vi "SL TAGS SystemLink Type To Class.vi"(8 "error in (no error)":errorcluster, 9 "SystemLink Cluster":T7, 11 "Class Tag In":T1={"Class Properties"={"Class Data Type"=enum."Double", "Name"="", "Description"="", "Interpolation Method"=enum."linear", "Unit of Measure"=enum."Hour", "Maximum Interpolation"="", "Role"=enum."Supervisor"}, "SL Tag"=refnum, "SystemLink Cluster"={"Path"="", "Data Type"=enum."Double", "Value"=variant, "Time Stamp"=timestamp(0 s since 1904-01-01)}, "Class Value"=variant}) -> (0 "error out":errorcluster, 3 "Class Tag Out":T1={"Class Properties"={"Class Data Type"=enum."Double", "Name"="", "Description"="", "Interpolation Method"=enum."linear", "Unit of Measure"=enum."Hour", "Maximum Interpolation"="", "Role"=enum."Supervisor"}, "SL Tag"=refnum, "SystemLink Cluster"={"Path"="", "Data Type"=enum."Double", "Value"=variant, "Time Stamp"=timestamp(0 s since 1904-01-01)}, "Class Value"=variant})   [LabVIEW 2017, in "EEISysLink.lvclass"]
doc: "At time of this library development SystemLink has mixed or no support for booleans & waveforms. This VI translates an extended set of data types in the class and more restricted in the SystemLink server from SystemLink type to class type.\n\nThis is a good location to seperate data types in SystemLink from those in the class. This allows the class to support any number of data types and translate to SystemLink types. This class translation is a good candidate for extending with additional data type classes to support an extended library functionality. \n\nJames Tillett P.E.\nEndeavor Engineering Inc.\nwww.endeavoreng.com"
uses:
  EEISysLink.lvclass
  <vilib>/Skyline/Tag/Shared/typedefs/Tag Cluster.ctl
  <vilib>/Skyline/Tag/Shared/typedefs/DataType.ctl
  Controls/SL Tag.ctl
  <vilib>/Skyline/Tag/Wrapper/Wrapper_class/NI Skyline Tag.lvclass
  Controls/SL Tag Properties.ctl
  Controls/SL Tag Data Type.ctl
  Controls/SL Tag Interpolation Method.ctl
  Controls/SL Tag Unit of Measure.ctl
  Controls/SL Tag Type.ctl
  Controls/SL Waveform.ctl
  <vilib>/Skyline/Tag/Shared/NI Skyline Tag.lvlib
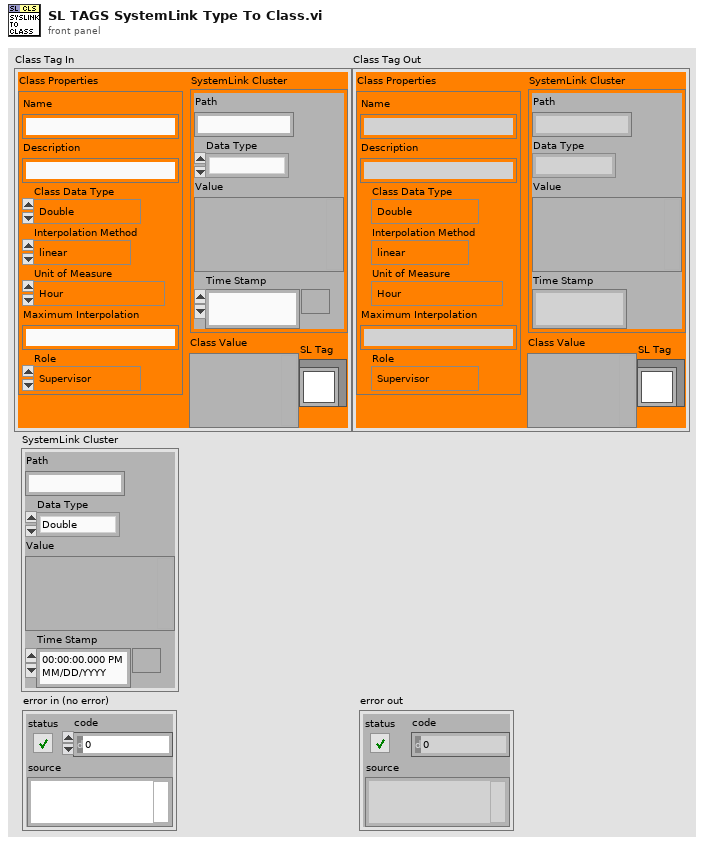
[diagram p1: front panel]
types:
  T1 = typedef "EEISysLink.lvclass/SL Tag.ctl" = cluster{"Class Properties":T2, "SL Tag":refnum<class "NI Skyline Tag.lvclass">, "SystemLink Cluster":T7, "Class Value":variant}
  T2 = typedef "EEISysLink.lvclass/SL Tag Properties.ctl" = cluster{"Class Data Type":T3, "Name":string, "Description":string, "Interpolation Method":T4, "Unit of Measure":T5, "Maximum Interpolation":string, "Role":T6}
  T3 = typedef "EEISysLink.lvclass/SL Tag Data Type.ctl" = enum16{"Double", "Integer", "String", "Boolean", "Waveform"}
  T4 = typedef "EEISysLink.lvclass/SL Tag Interpolation Method.ctl" = enum16{"linear", "pilinear", "step"}
  T5 = typedef "EEISysLink.lvclass/SL Tag Unit of Measure.ctl" = enum16{"no units", "Second", "Hour", "Minute", "Day", "Year", "Month", "Week", "Foot", "Yard", "Meter", "Centimeter", "Inch", "Mile", "Nautical Mile", "Miles per Hour", "Meters per second", "Square meter", "Cubic meter", "Cubic centimeter", "Cubic inch", "Liter", "Gallon", "Gallons dry US", "Gallon UK", "Percent", "Revolutions per minute", "Revolution", "Degree angle", "Astronomical Unit", "Atom", "Atomic mass", "Bar", "Byte", "C (speed of light)", "Curie", "Decibel", "Electron Volt", "Ounce", "Knot", "G", "Grade", "Are", "Hectare", "Faraday", "Franklin", "Gilbert", "Erg", "Lambert", "Maxwell", "Gauss", "Electron mass", "Kilogram force", "Pound force", "Rad", "Centiradian", "Sphere", "Mach", "Fluid Ounces", "Fluid Ounces UK", "Fahrenheit", "Celsius", "Kelvin", "Rankine", "Gram", "Kilogram", "Pound", "Short/US Ton", "Long/UK ton", "Metric ton", "Mole", "Pounds per square inch", "Inches water column", "Torr", "Millitorr", "Millimeter mercury", "Inches mercury", "Bar (2)", "Atmosphere", "Pascal", "Watt", "kiloWatt", "Horsepower", "Kilowatt Hour", "British thermal units", "Millions of BTU", "Ampere", "Candela", "Radian", "Steradian", "Bit", "Hertz", "Newton", "Joule", "Coulomb", "Volt", "Farad", "Ohm", "Siemens", "Weber", "Tesla", "Henry", "Lumen", "Lux", "Becqueral", "Gray", "Sievert", "Katal", "Angstrom", "Light Year", "Parsec", "Point", "Pixel", "Dyne", "Kilogram force (2)", "Pound force (2)", "Rem", "Rutherford", "Roentgen"}
  T6 = typedef "EEISysLink.lvclass/SL Tag Type.ctl" = enum16{"All", "Supervisor", "Worker"}
  T7 = typedef "NI Skyline Tag.lvlib/Tag Cluster.ctl" = cluster{"Path":string, "Data Type":T8, "Value":variant, "Time Stamp":timestamp}
  T8 = typedef "NI Skyline Tag.lvlib/DataType.ctl" = enum32{"Double", "Integer", "String"}
  T9 = typedef "EEISysLink.lvclass/SL Waveform.ctl" = cluster{"t0":dbl, "dt":dbl, "Y":dbl[]}
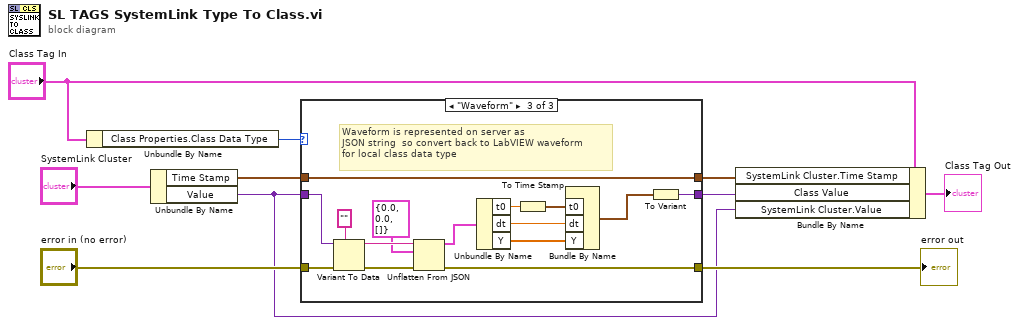
[diagram p0: block diagram]
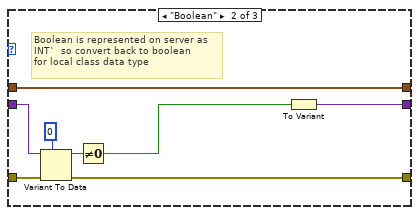
[diagram p3: hidden frame]
diagram:
  n1 = Unbundle By Name("Class Tag In") -> ("Class Properties.Class Data Type"=w10:T3)
  n2 = Unbundle By Name("SystemLink Cluster") -> ("Time Stamp"=w9:timestamp, "Value"=w1:variant)
  n3 = case shown="\"Waveform\"" w10 {
    tunnel: w9 -> [w13 w19 w35]
    tunnel: w1 -> [w12 w21 w36]
    tunnel: [w12 w20 w33] -> w5
    tunnel: [w13 w19 w35] -> w6
    tunnel: "error in (no error)" -> [w11 w18 w34]
    tunnel: [w11 w14 w22] -> w3
    frame Default {
      # "SystemLink supported so pass through unchanged"
    }
    frame "Boolean" {
      # "Boolean is represented on server as \nINT`  so convert back to boolean\nfor local class data type"
      n4 = Variant To Data(error in=w18, type=0, Variant=w21) -> (data=w16:i32, error out=w14:errorcluster)
      n5 = Not Equal To 0?(x=w16) -> (x != 0?=w15:bool)
      n6 = To Variant(anything=w15) -> (Variant=w20:variant)
    }
    frame "Waveform" {
      # "Waveform is represented on server as \nJSON string  so convert back to LabVIEW waveform\nfor local class data type"
      n7 = Variant To Data(error in=w34, type="", Variant=w36) -> (data=w30:string, error out=w31:errorcluster)
      n8 = Unflatten From JSON(JSON string=w30, type and defaults=T9 {"t0"=0.0, "dt"=0.0, "Y"=[]} ("SL Waveform"), error in (no error)=w31) -> (value=w28:T9, error out=w22:errorcluster)  [unwired: 4 in]
      n9 = Unbundle By Name(w28) -> ("t0"=w27:dbl, "dt"=w25:dbl, "Y"=w24:dbl[])
      n10 = To Time Stamp(1:w27) -> (0:w26:timestamp)
      n11 = Bundle By Name("t0"=w26, "dt"=w25, "Y"=w24) -> (w23:waveform(dbl))  [unwired: 1 in]
      n12 = To Variant(anything=w23) -> (Variant=w33:variant)
    }
  }
  "error out" <- w3
  n13 = Bundle By Name(cluster="Class Tag In", "SystemLink Cluster.Time Stamp"=w6, "Class Value"=w5, "SystemLink Cluster.Value"=w1) -> (→"Class Tag Out":T1)
